vi "Check.vi"() -> ()   [LabVIEW 2019]
uses:
  Z_source.ctl
  Z_HSw.lvclass
  Z_HSw.lvclass/Z_HSw.ctl
panel:
  in  "Z_Source":T1
  in  "connect":bool
  in  "stop":bool
  in  "Data":bool
  out "Z1 ind 3":u8(ring)
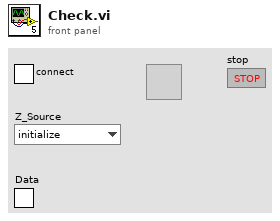
[diagram p1: front panel]
types:
  T1 = typedef "Z_source.ctl" = enum8{"initialize", "local disabled", "local hand", "hand", "auto", "dist"}
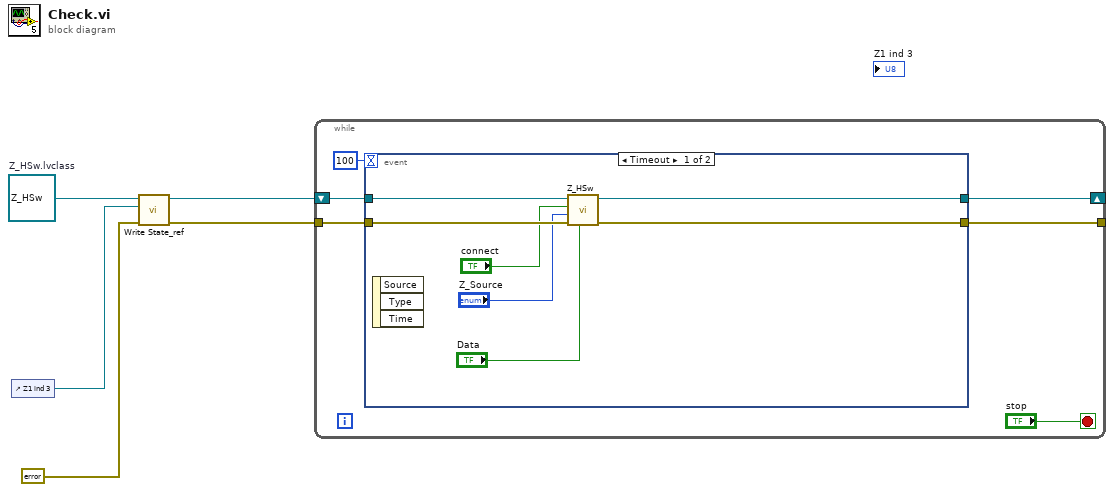
[diagram p0: block diagram]
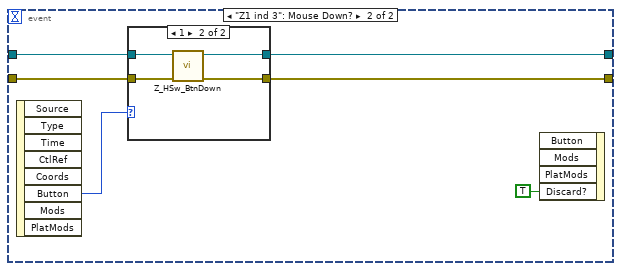
[diagram p2: hidden frame]
diagram:
  w5 = refnum<class "Z_HSw.lvclass"> refnum  # Z_HSw.lvclass
  n1 = control-ref of="Z1 ind 3"() -> (w4:refnum<vi>)
  n2 = call "Write State_ref.vi"("error in (no error)"=errorcluster {"status"=FALSE, "code"=0, "source"=""}, "State_ref"=w4, "Z_HSw in"=w5) -> ("error out"=w2:errorcluster, "Z_HSw out"=w3:refnum<class "Z_HSw.lvclass">)  [unwired: 7 in]
  n3 = while {
    tunnel: w2 -> [w7]
    shift-right: [w11] -> _
    shift-left: w3 -> [w9]
    tunnel: [w6] -> _
    stop <- "stop" stop-if-true
    n4 = event shown="[0] Timeout" {
      selector: _ -> [_ _]
      dyn-events: _ -> [_ _]
      timeout: 100 -> [_ _]
      tunnel: [w17 w22] -> w11
      tunnel: w9 -> [w16 w24]
      tunnel: w7 -> [w15 w23]
      tunnel: [w18 w21] -> w6
      event Timeout {
        n5 = event-data() -> ()  [unwired: 1 in, 3 out]
        n6 = call "Z_HSw.vi"("Data"="Data", "error in (no error)"=w15, "Z_Source"="Z_Source", "connect"="connect", "Z_HSw_in"=w16) -> ("error out"=w18:errorcluster, "Z_HSw_out"=w17:refnum<class "Z_HSw.lvclass">)  [unwired: 5 in]
      }
      event "Z1 ind 3": Mouse Down? {
        n7 = event-data() -> ("Button"=w20:u16)  [unwired: 1 in, 7 out]
        n8 = case shown="1" w20 {
          tunnel: w24 -> [w26 w30]
          tunnel: w23 -> [w25 w28]
          tunnel: [w26 w29] -> w22
          tunnel: [w25 w27] -> w21
          frame 0, Default {
          }
          frame 1 {
            n9 = call "Z_HSw_BtnDown.vi"("error in (no error)"=w28, "Z_HSw_in"=w30) -> ("error out"=w27:errorcluster, "Z_HSw_out"=w29:refnum<class "Z_HSw.lvclass">)  [unwired: 8 in]
          }
        }
        n10 = event-data("Discard?"=TRUE) -> ()  [unwired: 4 in, 1 out]
      }
    }
  }
